vi "_DServerStop.vi"(2 "error in":errorcluster, 3 "dserver evt.":T1) -> (0 "error out":errorcluster)   [LabVIEW 2014, in "tango.lvlib"]
uses:
  tango.lvlib
  Orphan/Typedefs/_DServerEvent.ctl
  Orphan/Typedefs/_DServerClientRequest.ctl
  Orphan/Typedefs/_DServerClientRequestType.ctl
  Orphan/Typedefs/_DServerClientRequestData.ctl
  Orphan/Typedefs/_GenericDataBuffer.ctl
  Orphan/Typedefs/_DataType.ctl
  tango_binding.so
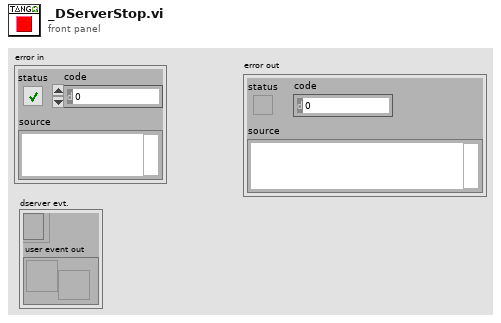
[diagram p1: front panel]
types:
  T1 = typedef "tango.lvlib/_DServerEvent.ctl" = cluster{"event registration refnum":refnum<event-registration>, "user event out":refnum<user-event>}
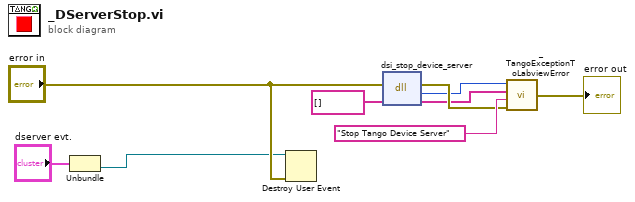
[diagram p0: block diagram]
diagram:
  n1 = Unbundle("dserver evt.") -> ("user event out"=w1:refnum<user-event>)  [unwired: 1 out]
  n2 = Destroy User Event(user event=w1, error in="error in") -> ()  [unwired: 1 out]
  n3 = dll-call lib="tango_binding.*" fn="dsi_stop_device_server"(error in="error in", "error_stack"=string[] [] ("error stack")) -> (error out=w8:errorcluster, "return type"=w6:i32, "error_stack"=w5:string[])  [unwired: 2 in, 1 out]
  n4 = call "_TangoExceptionToLabviewError.vi"("error in"=w8, "location"="Stop Tango Device Server", "error stack"=w5, "error code"=w6) -> ("error out"=→"error out":errorcluster)
